vi "Send Verify and Check-in.vi"(0 "Message Enqueuer":refnum<class "Message Enqueuer.lvclass">, 1 "Message Priority (Normal)":T1=enum."Normal", 5 "Room No":string, 7 "Guest Contact Number":string, 9 "Primary Guest Name":string, 11 "error in (no error)":errorcluster, 12 "Adults":u32, 13 "Children":u32) -> (4 "Message Enqueuer out":refnum<class "Message Enqueuer.lvclass">, 15 "error out":errorcluster)   [LabVIEW 2023, in "Incoming Rooms Manager Model Interface.lvlib" / "Verify and Check-in Msg.lvclass"]
doc: "This VI sends the message to an actor."
uses:
  Verify and Check-in Msg.lvclass
  Verify and Check-in Msg.lvclass/Verify and Check-in Msg.ctl
  <vilib>/ActorFramework/Message Enqueuer/Message Enqueuer.lvclass
  C:/Program Files/National Instruments/LabVIEW 2023/vi.lib/ActorFramework/Message/Message.lvclass
  C:/Users/bhaghyaraj/Trainings/NI Actor Framework/SDLC/Interfaces/Incoming Rooms Manager Model Interface Messages/Verify and Check-in Msg/Verify and Check-in Msg.lvclass
  <vilib>/ActorFramework/Message Enqueuer/Message Priority.ctl
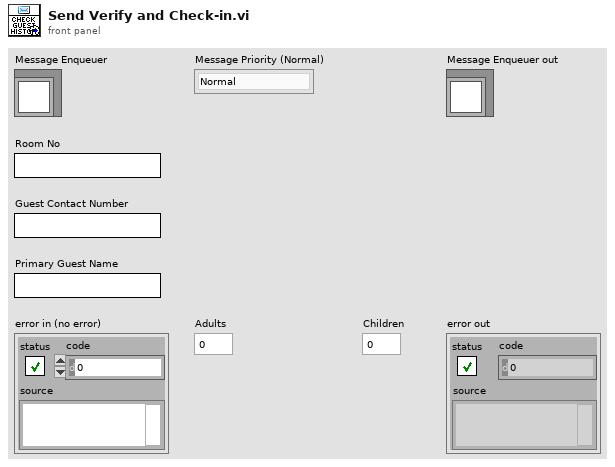
[diagram p1: front panel]
types:
  T1 = typedef "Actor Framework.lvlib/Message Enqueuer.lvclass/Message Priority.ctl" = enum16{"Low", "Normal", "High"}
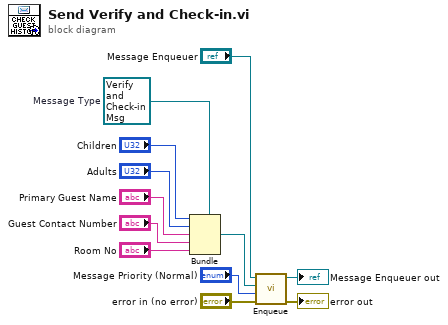
[diagram p0: block diagram]
diagram:
  w9 = refnum<class "Verify and Check-in Msg.lvclass"> refnum  # Message Type
  n1 = Bundle(cluster=w9, "Children", "Adults", "Primary Guest Name", "Guest Contact Number", "Room No") -> (w8:refnum<class "Verify and Check-in Msg.lvclass">)
  n2 = call <vilib>:"Enqueue.vi"("error in (no error)"="error in (no error)", "Message Priority (Normal)"="Message Priority (Normal)", "Message"=w8, "Message Enqueuer in"="Message Enqueuer") -> ("error out"=→"error out":errorcluster, "Message Enqueuer out"=→"Message Enqueuer out":refnum<class "Message Enqueuer.lvclass">)  [unwired: 6 in]
